vi "Test.vi"() -> ()   [LabVIEW 2018]
uses:
  phlib.dll
panel:
  out "Version 2":string
  out "return type":i32
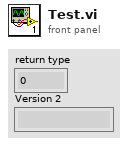
[diagram p1: front panel]
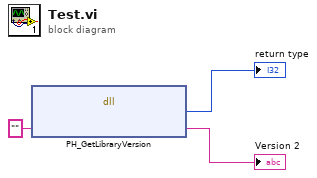
[diagram p0: block diagram]
diagram:
  n1 = dll-call lib="phlib.dll" fn="PH_GetLibraryVersion"("Version"="") -> ("return type"=→"return type":i32, "Version"=→"Version 2":string)  [unwired: 3 in, 2 out]
